vi "io_read.vi"(4 "Simulation read buffer (\"Simulation\")":string="Simulation", 5 "Trim Response (F)":bool, 6 "Block Logging (F)":bool, 8 "error in":errorcluster, 10 "byte count (2048)":u32=2048, 11 "VISA resource name":refnum<visa-resource-name>) -> (0 "error out":errorcluster, 1 "return count":u32, 2 "read buffer":string, 3 "VISA resource name out":refnum<visa-resource-name>)   [LabVIEW 2014, in "rszvl_rsidr_core.lvlib"]
uses:
  rszvl_rsidr_core.lvlib
  type_Error_Codes.ctl
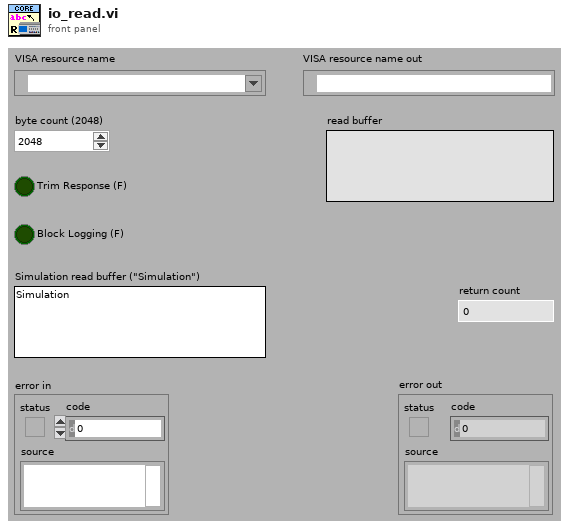
[diagram p1: front panel]
types:
  T1 = typedef "rszvl_rsidr_core.lvlib/type_Error_Codes.ctl" = enum16{"No_error", "VISA_err_ResourceNotFound", "VISA_err_Timeout", "VISA_warn_MoreDataAvailable", "RS_err_MissingCallback", "RS_err_InvalidAttribute", "RS_err_InvalidValue", "RS_err_UnknownResource", "RS_err_AlreadyInitialized", "RS_err_InstrumentStatus", "RS_err_BadRepCapName", "RS_err_TypesMismatch", "RS_err_ValueNotSupported", "RS_err_InvalidRngTable", "RS_err_IDqueryFail", "RS_err_UnexpResponse", "VISA_warn_ConfigNotLoaded", "RS_err_AttributeNotReadable", "RS_err_AttributeNotWritable", "RS_err_InstrumentType", "RS_err_InstrumentOption", "VISA_err_InvalidSize", "RS_err_ReliabilityIndicator", "VISA_warn_UnknownStatus", "VISA_warn_TermCharRead", "VISA_err_IO_error"}
  T2 = typedef "rszvl_rsidr_core.lvlib/type_Session_Data.ctl" = cluster{"Instr type":string, "Instr type for err. msg.":string, "Installed Options":string[], "OPC Timeout":i32, "Query Instrument Status":bool, "Check Range":bool, "Check Options":bool, "Add LF to Write":bool, "Simulate":bool, "Logging":bool, "Logging params":variant, "Interface Type":enum16{"Unknown", "GPIB", "VXI", "GPIB_VXI", "ASRL", "PXI", "TCPIP", "USB", "SOCKET"}, "Fast Sweep":i32, "AdditionalFlags":i32, "WaitBeforeWrite":i32, "WaitBeforeRead":i32, "BinDataChunkSize":i64}
  T3 = enum16{"Unknown", "GPIB", "VXI", "GPIB_VXI", "ASRL", "PXI", "TCPIP", "USB", "SOCKET"}
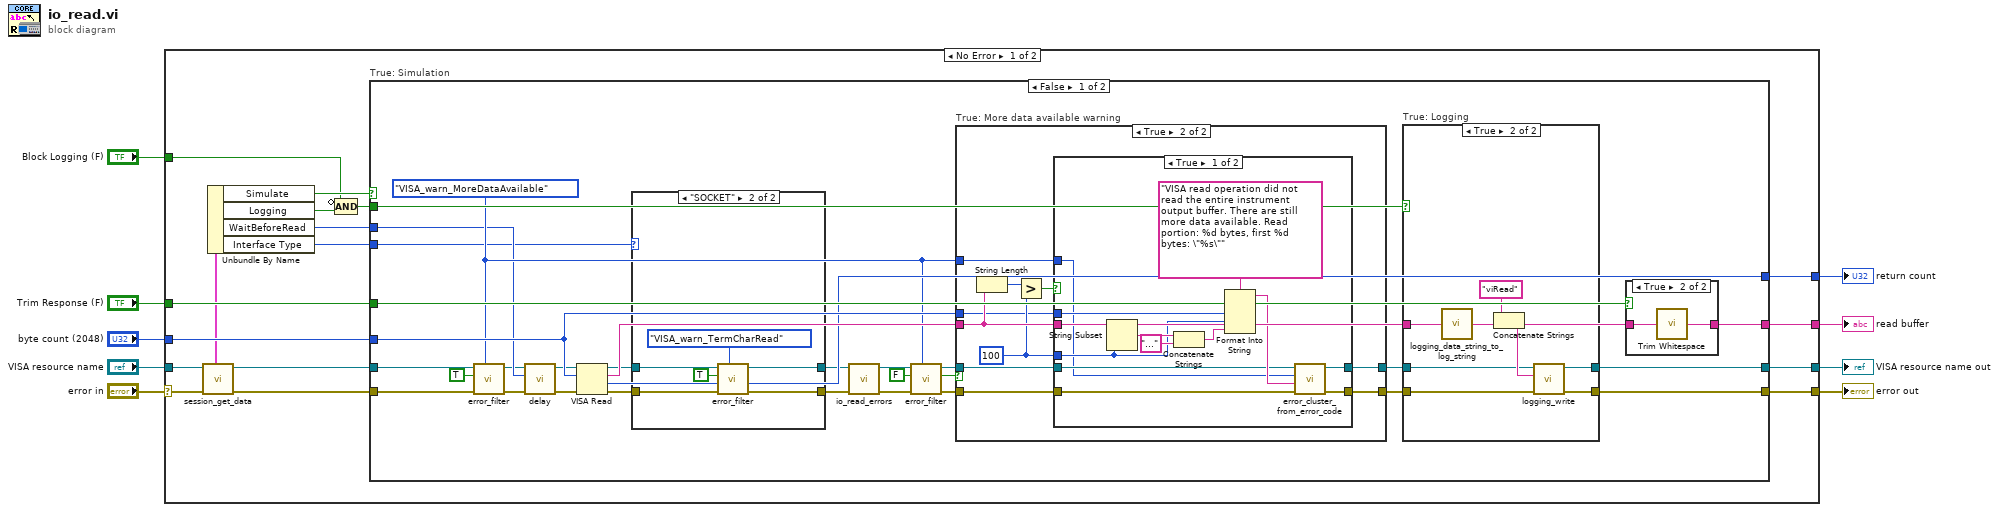
[diagram p0: block diagram]
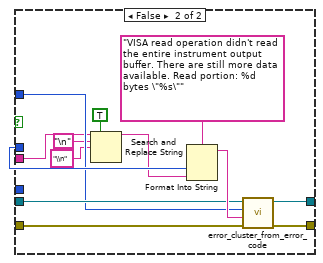
[diagram p5: hidden frame]
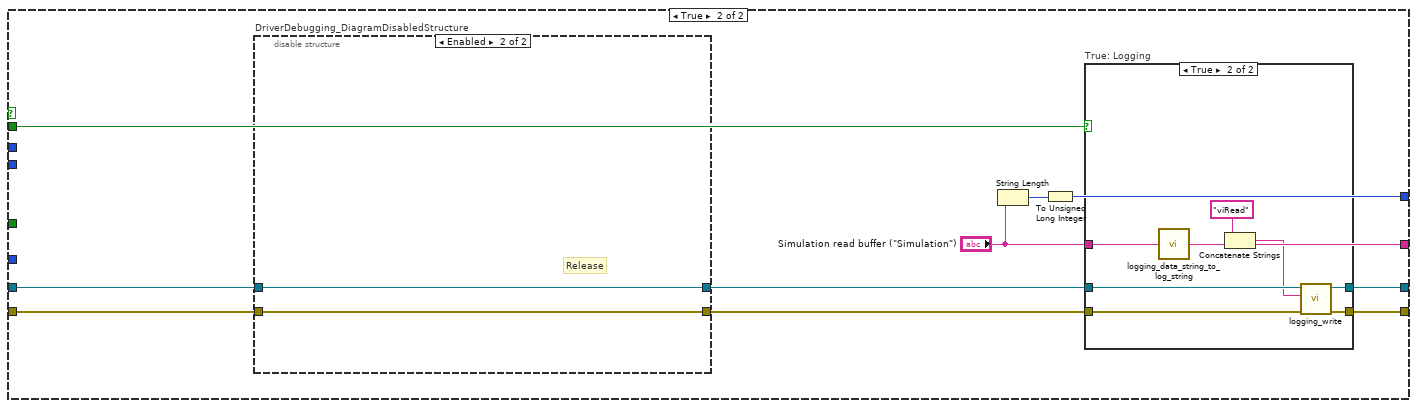
[diagram p7: hidden frame]
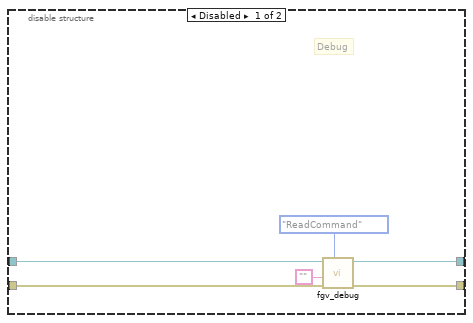
[diagram p8: hidden frame]
diagram:
  n1 = case shown="No Error" "error in" {
    selector: "error in" -> [w22 w145]
    tunnel: [w16 w145] -> w5
    tunnel: "byte count (2048)" -> [w26 _]
    tunnel: [w25 _] -> w8
    tunnel: "Trim Response (F)" -> [w24 _]
    tunnel: "VISA resource name" -> [w21 w144]
    tunnel: [w23 _] -> w6
    tunnel: [w15 w144] -> w4
    tunnel: "Block Logging (F)" -> [w10 _]
    frame No Error {
      n2 = call "session_get_data.vi"("error in"=w22, "VISA resource name"=w21) -> ("error out"=w20:errorcluster, "Session User Data out"=w18:T2, "VISA resource name out"=w19:refnum<visa-resource-name>)  [unwired: 7 in]
      n3 = Unbundle By Name(w18) -> ("Simulate"=w17:bool, "Logging"=w14:bool, "WaitBeforeRead"=w12:i32, "Interface Type"=w11:T3)
      n4 = Compound Arithmetic op=AND(invert w10, w14) -> (w13:bool)
      n5 = case "True: Simulation" shown="False" w17 {
        tunnel: [w56 w122] -> w16
        tunnel: w26 -> [w55 _]
        tunnel: [w53 "Simulation read buffer (\"Simulation\")"] -> w25
        tunnel: w24 -> [w52 _]
        tunnel: [w43 w120] -> w23
        tunnel: w20 -> [w42 w119]
        tunnel: w19 -> [w32 w117]
        tunnel: w13 -> [w50 w124]
        tunnel: [w51 w121] -> w15
        tunnel: w12 -> [w36 _]
        tunnel: w11 -> [w35 _]
        frame False {
          w41 = type_Error_Codes."VISA_warn_MoreDataAvailable" ("Code to detect")
          n6 = call "error_filter.vi"("Error Enum in"=w41, "error in"=w42, "Clear detected code (F)"=TRUE, "VISA resource name"=w32) -> ("error out"=w39:errorcluster, "VISA resource name out"=w31:refnum<visa-resource-name>)  [unwired: 5 in, 1 out]
          n7 = call "delay.vi"("error in"=w39, "Milliseconds to wait"=w36, "VISA resource name"=w31) -> ("error out"=w38:errorcluster, "VISA resource name out"=w37:refnum<visa-resource-name>)  [unwired: 7 in]
          n8 = VISA Read(VISA resource name=w37, byte count=w55, error in (no error)=w38) -> (VISA resource name out=w28:refnum<visa-resource-name>, read buffer=w54:string, return count=w43:u32, error out=w34:errorcluster)
          n9 = case shown="\"SOCKET\"" w35 {
            tunnel: w34 -> [w58 w64]
            tunnel: [w58 w62] -> w33
            tunnel: w28 -> [w57 w60]
            tunnel: [w57 w59] -> w27
            frame Default {
            }
            frame "SOCKET" {
              n10 = call "error_filter.vi"("Error Enum in"=type_Error_Codes."VISA_warn_TermCharRead" ("Code to detect"), "error in"=w64, "Clear detected code (F)"=TRUE, "VISA resource name"=w60) -> ("error out"=w62:errorcluster, "VISA resource name out"=w59:refnum<visa-resource-name>)  [unwired: 5 in, 1 out]
            }
          }
          n11 = call "io_read_errors.vi"("error in"=w33, "VISA resource name"=w27) -> ("error out"=w44:errorcluster, "VISA resource name out"=w30:refnum<visa-resource-name>)  [unwired: 8 in]
          n12 = call "error_filter.vi"("Error Enum in"=w41, "error in"=w44, "Clear detected code (F)"=FALSE ("Clear detected error (F)"), "VISA resource name"=w30) -> ("error out"=w48:errorcluster, "Code Detected"=w47:bool, "VISA resource name out"=w29:refnum<visa-resource-name>)  [unwired: 5 in]
          n13 = case "True: More data available warning" shown="True" w47 {
            tunnel: w48 -> [w76 w82]
            tunnel: [w76 w81] -> w46
            tunnel: w54 -> [_ w86]
            tunnel: w55 -> [_ w80]
            tunnel: w41 -> [_ w79]
            tunnel: w29 -> [w75 w78]
            tunnel: [w75 w77] -> w45
            frame False {
            }
            frame True {
              w84 = 100 ("length (rest)")
              n14 = String Length(string=w86) -> (length=w85:i32)
              n15 = Greater?(x=w85, y=w84) -> (0:w83:bool)
              n16 = case shown="True" w83 {
                tunnel: w86 -> [w99 w104]
                tunnel: w84 -> [w91 _]
                tunnel: w82 -> [w96 w112]
                tunnel: [w95 w111] -> w81
                tunnel: w80 -> [w93 w109]
                tunnel: w79 -> [w88 w105]
                tunnel: w78 -> [w90 w106]
                tunnel: [w89 w108] -> w77
                frame True {
                  n17 = String Subset(string=w99, length (rest)=w91) -> (substring=w98:string)  [unwired: 1 in]
                  n18 = Concatenate Strings(w98, "...") -> (w87:string)
                  n19 = Format Into String(format string="VISA read operation did not read the entire instrument output buffer. There are still more data available. Read portion: %d bytes, first %d bytes: \"%s\"", w93, w91, w87) -> (resulting string=w92:string)  [unwired: 2 in, 1 out]
                  n20 = call "error_cluster_from_error_code.vi"("error in"=w96, "error message (\"\")"=w92, "Error Enum in"=w88, "VISA resource name"=w90) -> ("error out"=w95:errorcluster, "VISA resource name out"=w89:refnum<visa-resource-name>)  [unwired: 6 in]
                }
                frame False {
                  n21 = Search and Replace String(replace all?=TRUE ("replace all? (F)"), input string=w104, search string="\n" ("Line Feed Constant"), replace string="\\n") -> (result string=w100:string)  [unwired: 4 in, 3 out]
                  n22 = Format Into String(format string="VISA read operation didn't read the entire instrument output buffer. There are still more data available. Read portion: %d bytes \"%s\"", w109, w100) -> (resulting string=w107:string)  [unwired: 2 in, 1 out]
                  n23 = call "error_cluster_from_error_code.vi"("error in"=w112, "error message (\"\")"=w107, "Error Enum in"=w105, "VISA resource name"=w106) -> ("error out"=w111:errorcluster, "VISA resource name out"=w108:refnum<visa-resource-name>)  [unwired: 6 in]
                }
              }
            }
          }
          n24 = case "True: Logging" shown="True" w50 {
            tunnel: w46 -> [w66 w74]
            tunnel: [w65 w73] -> w51
            tunnel: [w66 w72] -> w56
            tunnel: w54 -> [_ w71]
            tunnel: w45 -> [w65 w67]
            frame False {
            }
            frame True {
              n25 = call "logging_data_string_to_log_string.vi"("Raw string to log"=w71) -> ("Result log string"=w69:string)  [unwired: 4 in]
              n26 = Concatenate Strings("viRead" ("format string"), w69) -> (w68:string)
              n27 = call "logging_write.vi"("error in"=w74, "String to write"=w68, "VISA resource name"=w67) -> ("error out"=w72:errorcluster, "VISA resource name out"=w73:refnum<visa-resource-name>)  [unwired: 7 in]
            }
          }
          n28 = case shown="True" w52 {
            tunnel: w54 -> [w113 w115]
            tunnel: [w113 w114] -> w53
            frame False {
            }
            frame True {
              n29 = call "Trim Whitespace.vi"("string"=w115) -> ("trimmed string"=w114:string)  [unwired: 1 in]
            }
          }
        }
        frame True {
          n30 = disable-structure "DriverDebugging_DiagramDisabledStructure" shown="Enabled" {
            disable-tunnel: w119 -> [w131 w132]
            disable-tunnel: [w129 w132] -> w118
            disable-tunnel: w117 -> [w130 w133]
            disable-tunnel: [w128 w133] -> w116
            frame Disabled {
              # "Debug"
              n31 = call "fgv_debug.vi"("Operation"=enum16{"Reset", "ReadCommand", "SetCommand"}."ReadCommand", "error in"=w131, "Command in"="" ("Empty String Constant"), "VISA resource name"=w130) -> ("error out"=w129:errorcluster, "VISA resource name out"=w128:refnum<visa-resource-name>)  [unwired: 6 in]
            }
            frame Enabled {
              # "Release"
            }
          }
          n32 = String Length(string="Simulation read buffer (\"Simulation\")") -> (length=w125:i32)
          n33 = To Unsigned Long Integer(number=w125) -> (unsigned 32bit integer=w120:u32)
          n34 = case "True: Logging" shown="True" w124 {
            tunnel: "Simulation read buffer (\"Simulation\")" -> [_ w139]
            tunnel: w118 -> [w135 w143]
            tunnel: w116 -> [w134 w142]
            tunnel: [w135 w141] -> w122
            tunnel: [w134 w140] -> w121
            frame False {
            }
            frame True {
              n35 = call "logging_data_string_to_log_string.vi"("Raw string to log"=w139) -> ("Result log string"=w138:string)  [unwired: 4 in]
              n36 = Concatenate Strings("viRead" ("format string"), w138) -> (w137:string)
              n37 = call "logging_write.vi"("error in"=w143, "String to write"=w137, "VISA resource name"=w142) -> ("error out"=w141:errorcluster, "VISA resource name out"=w140:refnum<visa-resource-name>)  [unwired: 7 in]
            }
          }
        }
      }
    }
    frame Error {
    }
  }
  "VISA resource name out" <- w4
  "error out" <- w5
  "read buffer" <- w8
  "return count" <- w6
